vi "FL_Decode_RAW_to_DEC_last_out.vi"(3 "Input array of timestamps":timestamp[](array[timestamp]), 4 "Half-height of the sensor board":sgl=125.0, 5 "Half-width of the sensor board":sgl=137.5, 6 "Sensors grid step":sgl=25.0, 7 "read buffer":string) -> (0 "Output timestamp":timestamp, 1 "DEC output":sgl[](array[numeric]))   [LabVIEW 2016]
panel:
  out "offset past match":i32
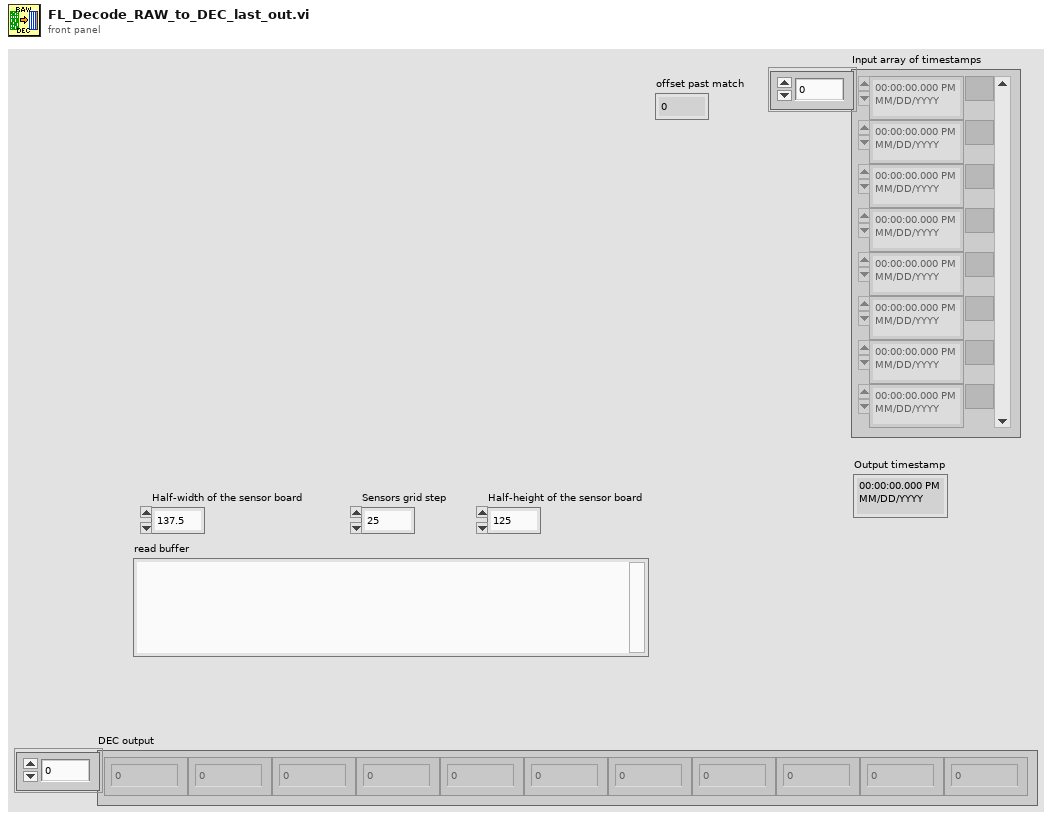
[diagram p1: front panel]
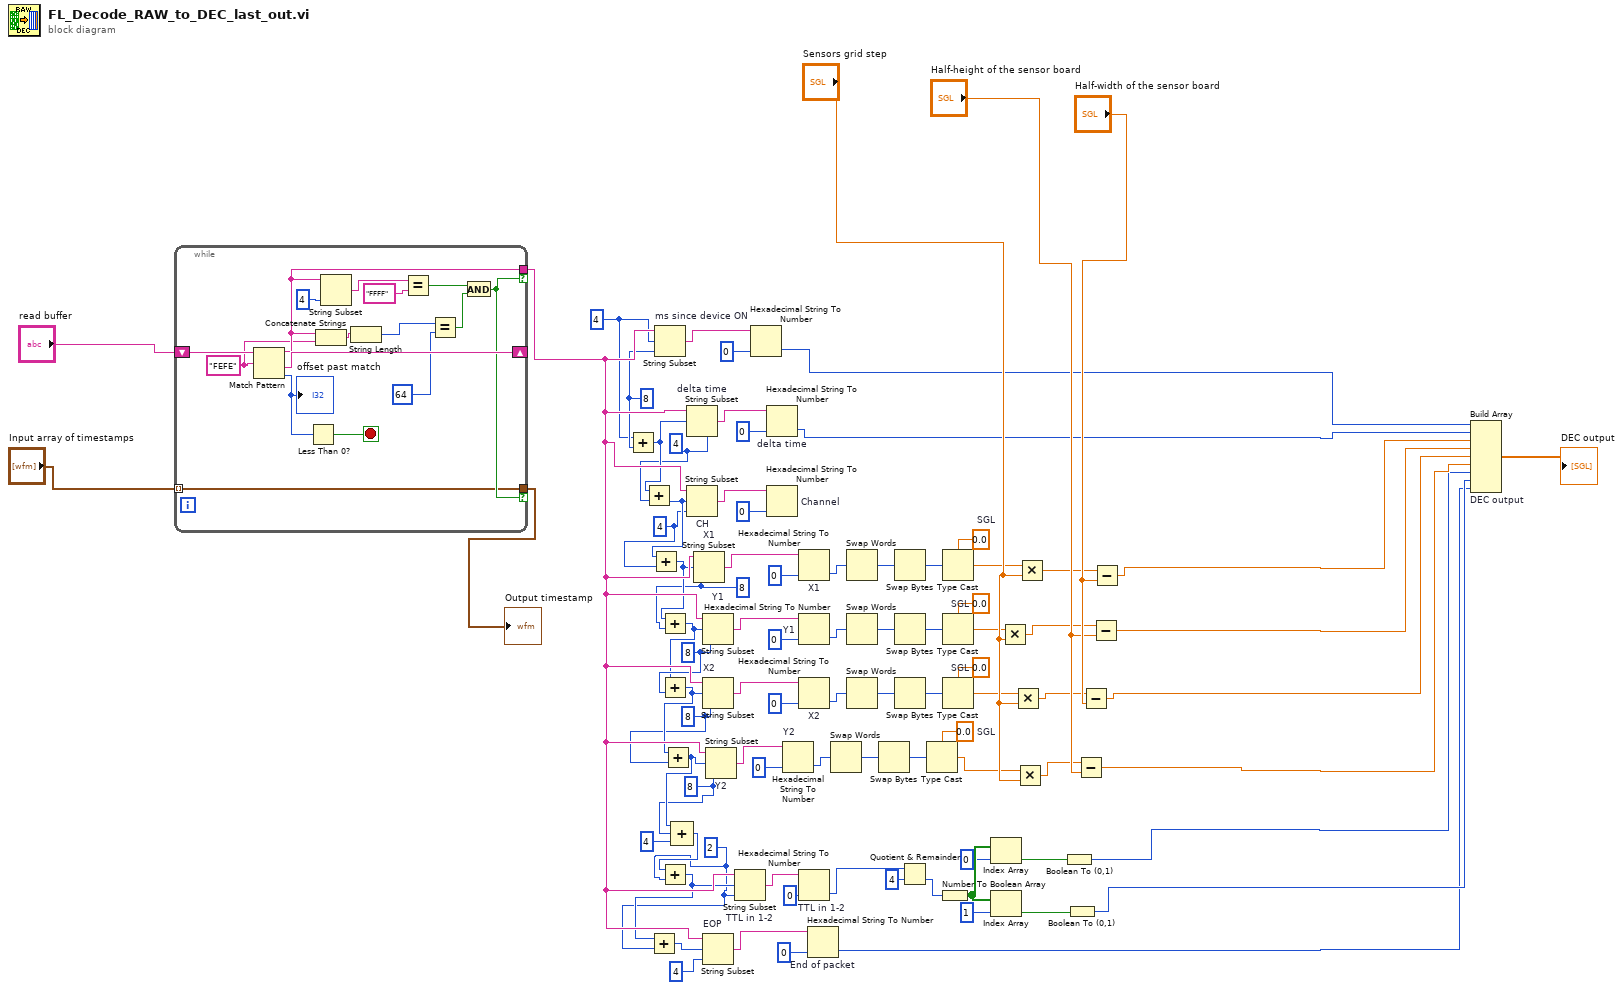
[diagram p0: block diagram]
diagram:
  w3 = 4
  w13 = 2 ("length (rest)")
  w29 = sgl 0.0  # SGL
  w36 = sgl 0.0  # SGL
  w43 = sgl 0.0  # SGL
  w49 = sgl 0.0  # SGL
  w18 = 8 ("length (rest)")
  w62 = 8 ("length (rest)")
  w65 = 8 ("length (rest)")
  w66 = 8 ("length (rest)")
  w68 = 4 ("length (rest)")
  w70 = 4 ("length (rest)")
  w72 = 8 ("length (rest)")
  n1 = while {
    shift-right: [w102] -> _
    shift-left: "read buffer" -> [w103]
    tunnel: [w92] -> w86 if=w89
    tunnel: [w88] -> w1 if=w89
    tunnel: "Input array of timestamps" -> [w88] mode=indexing
    stop <- w100 stop-if-true
    w90 = "FEFE" ("regular expression")
    n2 = Match Pattern(string=w103, regular expression=w90) -> (before substring=w92:string, after substring=w102:string, offset past match=w101:i32)  [unwired: 1 in, 1 out]
    "offset past match" <- w101
    n3 = Less Than 0?(x=w101) -> (x < 0?=w100:bool)
    n4 = Concatenate Strings(w92, w90) -> (w91:string)
    n5 = String Subset(string=w92, length (rest)=4 ("length (rest)")) -> (substring=w98:string)  [unwired: 1 in]
    n6 = String Length(string=w91) -> (length=w96:i32)
    n7 = Equal?(x=w98, y="FFFF") -> (x = y?=w94:bool)
    n8 = Equal?(x=w96, y=64) -> (x = y?=w93:bool)
    n9 = And(x=w94, y=w93) -> (x .and. y?=w89:bool)
  }
  "Output timestamp" <- w1
  n10 = Add(x=w3, y=w72) -> (x+y=w71:i32)
  n11 = Add(x=w71, y=w70) -> (x+y=w69:i32)
  n12 = Add(x=w69, y=w68) -> (x+y=w67:i32)
  n13 = String Subset "ms since device ON"(string=w86, offset (0)=w3, length (rest)=w72) -> (substring=w59:string)
  n14 = Add(x=w67, y=w66) -> (x+y=w64:i32)
  n15 = Add(x=w64, y=w65) -> (x+y=w63:i32)
  n16 = Add(x=w63, y=w62) -> (x+y=w19:i32)
  n17 = Compound Arithmetic op=unknown(w19, w18, 4 ("value")) -> (w15:i32)
  n18 = Add(x=w15, y=w13) -> (x+y=w14:i32)
  n19 = Add(x=w14, y=w13) -> (x+y=w61:i32)
  n20 = String Subset "delta time"(string=w86, offset (0)=w71, length (rest)=w70) -> (substring=w56:string)
  n21 = String Subset "CH"(string=w86, offset (0)=w69, length (rest)=w68) -> (substring=w54:string)
  n22 = String Subset "X1"(string=w86, offset (0)=w67, length (rest)=w66) -> (substring=w53:string)
  n23 = String Subset "Y1"(string=w86, offset (0)=w64, length (rest)=w65) -> (substring=w41:string)
  n24 = String Subset "X2"(string=w86, offset (0)=w63, length (rest)=w62) -> (substring=w34:string)
  n25 = String Subset "EOP"(string=w86, offset (0)=w61, length (rest)=4 ("length (rest)")) -> (substring=w24:string)
  n26 = String Subset "Y2"(string=w86, offset (0)=w19, length (rest)=w18) -> (substring=w27:string)
  n27 = String Subset "TTL in 1-2"(string=w86, offset (0)=w14, length (rest)=w13) -> (substring=w17:string)
  n28 = Hexadecimal String To Number ("ms since ON")(string=w59, default (0uL)=u32 0 ("default (0 U32)")) -> (number=w81:u32)  [unwired: 1 in, 1 out]
  n29 = Hexadecimal String To Number "delta time"(string=w56, default (0uL)=u32 0 ("default (0 U32)")) -> (number=w80:u32)  [unwired: 1 in, 1 out]
  n30 = Hexadecimal String To Number "Channel"(string=w54, default (0uL)=u32 0 ("default (0 U32)")) -> ()  [unwired: 1 in, 2 out]
  n31 = Hexadecimal String To Number "Y2"(string=w27, default (0uL)=u32 0 ("default (0 U32)")) -> (number=w31:u32)  [unwired: 1 in, 1 out]
  n32 = Hexadecimal String To Number "X1"(string=w53, default (0uL)=u32 0 ("default (0 U32)")) -> (number=w51:u32)  [unwired: 1 in, 1 out]
  n33 = Hexadecimal String To Number "Y1"(string=w41, default (0uL)=u32 0 ("default (0 U32)")) -> (number=w45:u32)  [unwired: 1 in, 1 out]
  n34 = Hexadecimal String To Number "X2"(string=w34, default (0uL)=u32 0 ("default (0 U32)")) -> (number=w38:u32)  [unwired: 1 in, 1 out]
  n35 = Hexadecimal String To Number "TTL in 1-2"(string=w17, default (0uL)=u32 0 ("default (0 U32)")) -> (number=w10:u32)  [unwired: 1 in, 1 out]
  n36 = Hexadecimal String To Number "End of packet"(string=w24, default (0uL)=u32 0 ("default (0 U32)")) -> (number=w73:u32)  [unwired: 1 in, 1 out]
  n37 = Swap Words(1:w31) -> (0:w30:u32)
  n38 = Swap Words(1:w51) -> (0:w50:u32)
  n39 = Swap Words(1:w45) -> (0:w44:u32)
  n40 = Swap Words(1:w38) -> (0:w37:u32)
  n41 = Swap Bytes(anything=w30) -> (byte swapped=w28:u32)
  n42 = Swap Bytes(anything=w50) -> (byte swapped=w48:u32)
  n43 = Swap Bytes(anything=w44) -> (byte swapped=w42:u32)
  n44 = Swap Bytes(anything=w37) -> (byte swapped=w35:u32)
  n45 = Quotient & Remainder(x=w10, y=u32 4) -> (floor(x/y)=w9:u32)  [unwired: 1 out]
  n46 = Type Cast(type=w29, x=w28) -> (*(type *) &x=w26:sgl)
  n47 = Number To Boolean Array(number=w9) -> (Boolean array=w8:bool[])
  n48 = Type Cast(type=w49, x=w48) -> (*(type *) &x=w47:sgl)
  n49 = Type Cast(type=w43, x=w42) -> (*(type *) &x=w40:sgl)
  n50 = Type Cast(type=w36, x=w35) -> (*(type *) &x=w33:sgl)
  n51 = Index Array(array=w8, index=0) -> (element=w5:bool)
  n52 = Index Array(array=w8, index=1) -> (element=w4:bool)
  n53 = Multiply(x=w40, y="Sensors grid step") -> (x*y=w21:sgl)
  n54 = Multiply(x=w33, y="Sensors grid step") -> (x*y=w22:sgl)
  n55 = Multiply(x=w26, y="Sensors grid step") -> (x*y=w20:sgl)
  n56 = Multiply(x=w47, y="Sensors grid step") -> (x*y=w23:sgl)
  n57 = Boolean To (0,1)(Boolean=w5) -> (0, 1=w75:i16)
  n58 = Boolean To (0,1)(Boolean=w4) -> (0, 1=w74:i16)
  n59 = Subtract(x=w20, y="Half-height of the sensor board") -> (x-y=w76:sgl)
  n60 = Subtract(x=w22, y="Half-width of the sensor board") -> (x-y=w77:sgl)
  n61 = Subtract(x=w21, y="Half-height of the sensor board") -> (x-y=w78:sgl)
  n62 = Subtract(x=w23, y="Half-width of the sensor board") -> (x-y=w79:sgl)
  n63 = Build Array "DEC output"(w81, w80, w79, w78, w77, w76, w75, w74, w73) -> (→"DEC output":sgl[])
